vi "Set Motor Type.vi"(4 "Motor Type (Undefined)":T1(ring), 5 "error in (no error)":errorcluster, 7 "Axis (1)":i32=1 min=1 max=3, 8 "VISA resource name":refnum<visa-resource-name>) -> (0 "error out":errorcluster, 3 "VISA resource name out":refnum<visa-resource-name>)   [LabVIEW 2014, in "Newport ESP301.lvlib"]
doc: "This command is used to set the motor type the for axis <B>Axis (1)</B>. Defining motor type is necessary because the ESP needs to apply different control algorithms for different motor types.\n<B>NOTE:</B> It will not be possible to control an axis if its motor type is undefined."
uses:
  Newport ESP301.lvlib
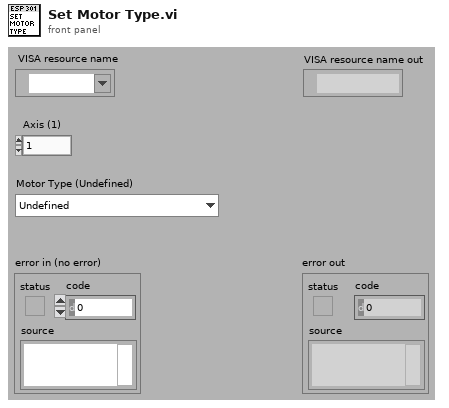
[diagram p1: front panel]
types:
  T1 = enum16{"Undefined", "DC Servo Motor", "Step Motor (not supported)", "Commutated Step Motor", "Commutate Brushless DC Servo Motor"}
  T2 = enum16{"Undefined", "DC Servo Motor", "Step Motor", "Commutated Step Motor (not supported)", "Commutate Brushless DC Servo Motor"}
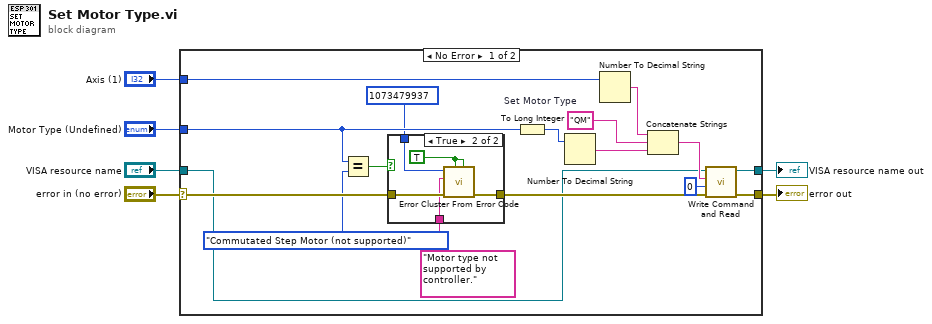
[diagram p0: block diagram]
diagram:
  n1 = case shown="No Error" "error in (no error)" {
    selector: "error in (no error)" -> [w14 w31]
    tunnel: [w23 w31] -> w5
    tunnel: "VISA resource name" -> [w7 w30]
    tunnel: [w22 w30] -> w3
    tunnel: "Axis (1)" -> [w18 _]
    tunnel: "Motor Type (Undefined)" -> [w10 _]
    frame No Error {
      w20 = "QM"  # Set Motor Type
      n2 = Equal?(x=w10, y=T2."Commutated Step Motor (not supported)" ("Motor Type (Undefined) 2")) -> (x = y?=w12:bool)
      n3 = case shown="True" w12 {
        tunnel: w14 -> [w24 w29]
        tunnel: [w24 w28] -> w13
        tunnel: 1073479937 -> [_ w27]
        tunnel: "Motor type not supported by controller." -> [_ w25]
        frame False {
        }
        frame True {
          w26 = TRUE ("show call chain? (False)")
          n4 = call <vilib>:"Error Cluster From Error Code.vi"("is warning? (False)"=w26, "show call chain? (False)"=w26, "error in (no error)"=w29, "error message (\"\")"=w25, "error code (0)"=w27) -> ("error out"=w28:errorcluster)  [unwired: 4 in]
        }
      }
      n5 = To Long Integer(number=w10) -> (32bit integer=w15:i32)
      n6 = Number To Decimal String(number=w15) -> (decimal integer string=w21:string)  [unwired: 1 in]
      n7 = Number To Decimal String(number=w18) -> (decimal integer string=w19:string)  [unwired: 1 in]
      n8 = Concatenate Strings(w19, w20, w21) -> (w17:string)
      n9 = call "Write Command and Read.vi"("error in (no error)"=w13, "Bytes to read (100)"=u32 0, "Command"=w17, "VISA resource name"=w7) -> ("error out"=w23:errorcluster, "VISA resource name out"=w22:refnum<visa-resource-name>)  [unwired: 3 in, 1 out]
    }
    frame Error {
    }
  }
  "error out" <- w5
  "VISA resource name out" <- w3
